vi "programacion 11 Lester Roche.vi"() -> ()   [LabVIEW 2011]
uses:
  <vilib>/express/express arith-compare/Formula/XNode/ExpressFormulaBlockNode.xnode
panel:
  out "Menor":dbl
  out "Mayor":dbl
  out "Promedio":dbl
  out "Contador":dbl
  out "Numeros Par":dbl
  # "Elaborar un programa donde se generen y presenten 5\nnumeros pares. Obtener el promedio, el numero mayor y menor."
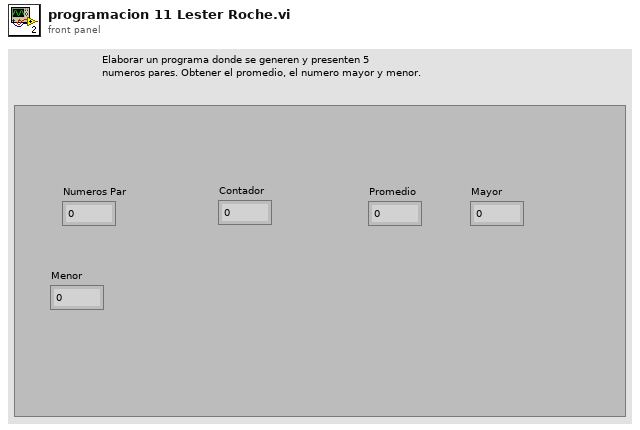
[diagram p1: front panel]
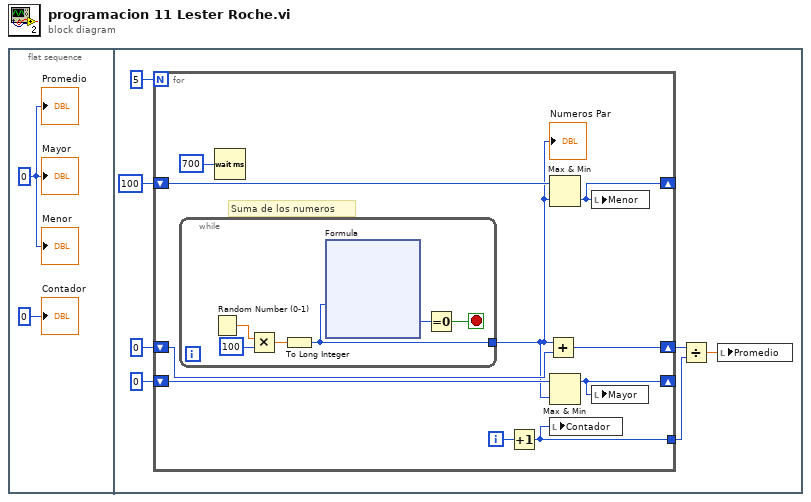
[diagram p0: block diagram]
diagram:
  n1 = flat-sequence {
    frame #0 {
      w1 = 0
      "Contador" <- 0
      "Menor" <- w1
      "Promedio" <- w1
      "Mayor" <- w1
    }
    frame #1 {
      n2 = for {
        N: 5 -> [_]
        shift-right: [w16] -> w7
        shift-left: 0 -> [w17]
        tunnel: [w15] -> w6
        shift-right: [w11] -> _
        shift-left: 0 -> [w14]
        shift-right: [w10] -> _
        shift-left: 100 -> [w13]
        i -> [w19]
        # "Suma de los numeros"
        n3 = while {
          tunnel: [w20] -> w12
          stop <- w21 stop-if-true
          n4 = Random Number (0-1)() -> (number: 0 to 1=w25:dbl)
          n5 = Multiply(x=w25, y=100) -> (x*y=w23:dbl)
          n6 = To Long Integer(number=w23) -> (32bit integer=w20:i32)
          n7 = xnode "Formula"("X1"=w20) -> ("Result"=w22:i32)  [unwired: 1 in, 1 out]
          n8 = Equal To 0?(x=w22) -> (x = 0?=w21:bool)
        }
        "Numeros Par" <- w12
        n9 = Wait (ms)(milliseconds to wait=700) -> ()  [unwired: 1 out]
        n10 = Increment(x=w19) -> (x+1=w15:i32)
        n11 = Add(x=w12, y=w17) -> (x+y=w16:i32)
        n12 = Max & Min(x=w13, y=w12) -> (min(x,y)=w10:i32)  [unwired: 1 out]
        n13 = Max & Min(x=w14, y=w12) -> (max(x,y)=w11:i32)  [unwired: 1 out]
        n14 = local write "Contador"(w15) -> ()
        n15 = local write "Menor"(w10) -> ()
        n16 = local write "Mayor"(w11) -> ()
      }
      n17 = Divide(x=w7, y=w6) -> (x/y=w5:dbl)
      n18 = local write "Promedio"(w5) -> ()
    }
  }
